vi "next field-subvi.vi"(8 "Error In":errorcluster) -> (0 "Error Out":errorcluster)   [LabVIEW 2014]
doc: "Increments the field number on stage-controller.vi by one. The number of times this VI is called is determined by Max Cycles in multi-mode-acquisition.vi."
uses:
  ctts/move stage.ctl
  stage-controller-globals.vi
panel:
  out "Current Field Size":i32
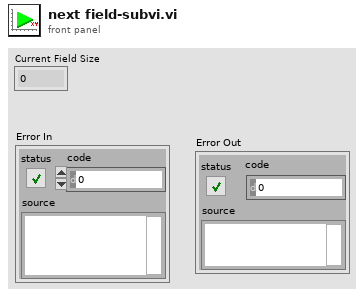
[diagram p1: front panel]
types:
  T1 = typedef "move stage.ctl" = cluster{"dx (um) (0 -> ignore)":ext, "dy (um) (0 -> ignore)":ext, "dz (um) (0 -> ignore)":ext, "Re-center x,y":bool, "Re-center z":bool, "x (um) (-1 -> ignore)":dbl, "y (um) (-1 -> ignore)":dbl, "z (um) (-1 -> ignore)":dbl, "Move to Next Field":bool}
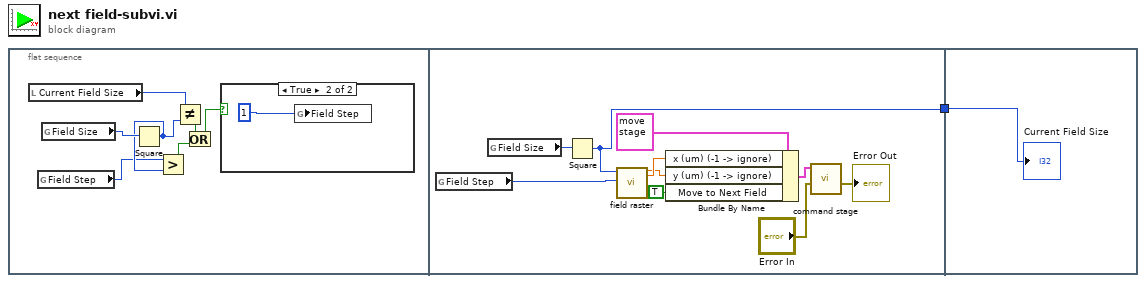
[diagram p0: block diagram]
diagram:
  n1 = flat-sequence {
    tunnel: [w11] -> w1
    tunnel: w1 -> [w20]
    frame #0 {
      n2 = local read "Current Field Size"() -> (w7:i32)
      n3 = global read "stage-controller-globals.vi" "Field Step"() -> (w2:u32)
      n4 = global read "stage-controller-globals.vi" "Field Size"() -> (w8:enum16{"0", "1", "4", "9", "16"})
      n5 = Square(x=w8) -> (x^2=w3:u16)
      n6 = Greater?(x=w2, y=w3) -> (0:w4:bool)
      n7 = Not Equal?(x=w7, y=w3) -> (x != y?=w6:bool)
      n8 = Or(x=w6, y=w4) -> (x .or. y?=w5:bool)
      n9 = case shown="True" w5 {
        frame False {
        }
        frame True {
          n10 = global write "stage-controller-globals.vi" "Field Step"(1) -> ()
        }
      }
    }
    frame #1 {
      n11 = global read "stage-controller-globals.vi" "Field Step"() -> (w14:u32)
      n12 = global read "stage-controller-globals.vi" "Field Size"() -> (w19:enum16{"0", "1", "4", "9", "16"})
      n13 = Square(x=w19) -> (x^2=w11:u16)
      n14 = call "field raster.vi"("field size"=w11, "field number"=w14) -> ("current Y"=w12:dbl, "current X"=w13:dbl)  [unwired: 12 in, 4 out]
      n15 = Bundle By Name(cluster=T1 {"dx (um) (0 -> ignore)"=0.0, "dy (um) (0 -> ignore)"=0.0, "dz (um) (0 -> ignore)"=0.0, "Re-center x,y"=FALSE, "Re-center z"=FALSE, "x (um) (-1 -> ignore)"=-1.0, "y (um) (-1 -> ignore)"=-1.0, "z (um) (-1 -> ignore)"=-1.0, "Move to Next Field"=FALSE} ("Move stage\ncommand"), "x (um) (-1 -> ignore)"=w13, "y (um) (-1 -> ignore)"=w12, "Move to Next Field"=TRUE) -> (w16:T1)
      n16 = call "command stage.vi"("Error In"="Error In", "Command Stage"=w16) -> ("Error Out"=→"Error Out":errorcluster)  [unwired: 9 in]
    }
    frame #2 {
      "Current Field Size" <- w20
    }
  }
